vi "Do.vi"(8 "error in (no error)":errorcluster, 10 "Actor in":refnum<class "Actor.lvclass">, 11 "FlushAppenderMsg":refnum<class "FlushAppenderMsg.lvclass">) -> (0 "error out":errorcluster, 2 "Actor out":refnum<class "Actor.lvclass">)   [LabVIEW 2026, in "Lumberjack.lvlib" / "FlushAppenderMsg.lvclass"]
doc: "<p>(<strong>Filename</strong>: <span class=\"dnl\">Actor Framework.lvlib:Message.lvclass:Do.vi</span>)</p>\n<p>Defines what a message does when it is received by an actor. Generally, a message instructs an actor to invoke one of its methods. By default, this method does nothing. A child class must override it to define behavior.</p>"
uses:
  FlushAppenderMsg.lvclass
  <vilib>/ActorFramework/Actor/Actor.lvclass
  Appenders/Appender.lvclass/Appender.lvclass
  C:/Program Files (x86)/National Instruments/LabVIEW 2026/vi.lib/ActorFramework/Actor/Actor.lvclass
  FlushAppenderMsg.lvclass/FlushAppenderMsg.ctl
  FlushAckMsg.lvclass/FlushAckMsg.lvclass
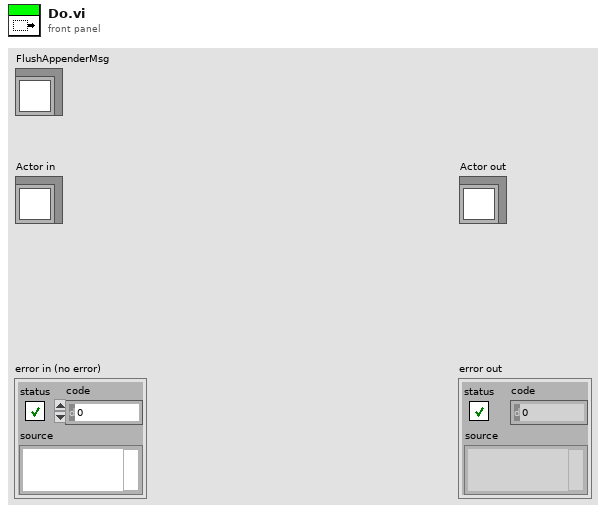
[diagram p1: front panel]
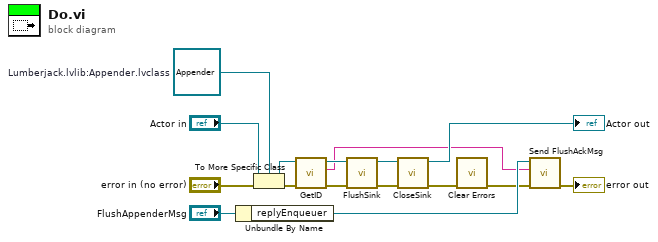
[diagram p0: block diagram]
diagram:
  w14 = refnum<class "Appender.lvclass"> refnum  # Lumberjack.lvlib:Appender.lvclass
  n1 = Unbundle By Name("FlushAppenderMsg") -> ("replyEnqueuer"=w12:refnum<class "Message Enqueuer.lvclass">)
  n2 = To More Specific Class(target class=w14, reference="Actor in", error in="error in (no error)") -> (specific class reference=w11:refnum<class "Appender.lvclass">, error out=w10:errorcluster)
  n3 = call "GetID.vi"("error in (no error)"=w10, "Appender in"=w11) -> ("error out"=w9:errorcluster, "ID"=w1:string, "Appender out"=w8:refnum<class "Appender.lvclass">)  [unwired: 7 in]
  n4 = call-dynamic "FlushSink.vi"("error in (no error)"=w9, "Appender in"=w8) -> ("error out"=w4:errorcluster, "Appender out"=w7:refnum<class "Appender.lvclass">)  [unwired: 8 in]
  n5 = call-dynamic "CloseSink.vi"("error in (no error)"=w4, "Appender in"=w7) -> ("error out"=w3:errorcluster, "Appender out"=→"Actor out":refnum<class "Appender.lvclass">)  [unwired: 8 in]
  n6 = call <vilib>:"Clear Errors.vi"("error in (no error)"=w3) -> ("error out"=w5:errorcluster)  [unwired: 5 in, 1 out]
  n7 = call "Send FlushAckMsg.vi"("error in (no error)"=w5, "appenderID"=w1, "Enqueuer in"=w12) -> ("error out"=→"error out":errorcluster)  [unwired: 7 in, 1 out]
